vi "Init Power Meter.vi"(8 "error in (no error)":errorcluster, 11 "Application in":refnum<class "Application.lvclass">) -> (0 "error out":errorcluster, 3 "Application out":refnum<class "Application.lvclass">)   [LabVIEW 2018, in "Application.lvlib" / "Application.lvclass"]
uses:
  Application.lvclass
  C:/Program Files/National Instruments/LabVIEW 2018/vi.lib/ActorFramework/Actor/Actor.lvclass
  Application.lvclass/Application.ctl
  User Interface/Splash Screen Messages/Update Status Msg/Update Status Msg.lvclass/Update Status Msg.ctl
  <vilib>/ActorFramework/Message Enqueuer/Message Enqueuer.lvclass/Message Enqueuer.ctl
  <vilib>/ActorFramework/Message Enqueuer/Enqueue.vi
  User Interface/Splash Screen Messages/Update Status Msg/Update Status Msg.lvclass
  C:/Program Files/National Instruments/LabVIEW 2018/vi.lib/ActorFramework/Message/Message.lvclass
  Hardware/Power Meter/Power Meter/Power Meter.lvclass
  <vilib>/ActorFramework/Message Priority Queue/Priority Enqueue.vi
  <vilib>/ActorFramework/Actor/Actor.lvclass
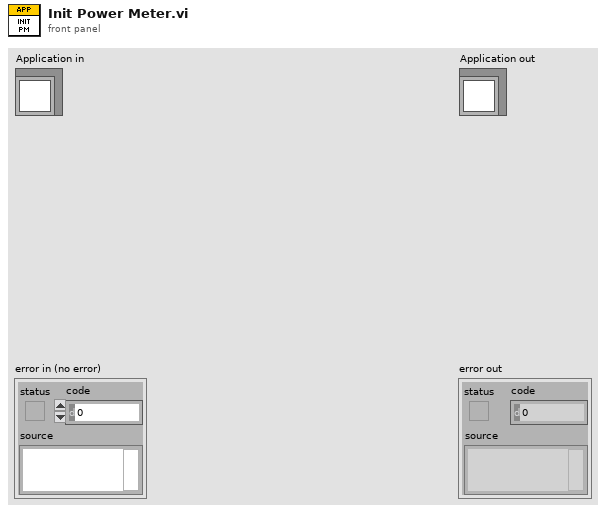
[diagram p1: front panel]
types:
  T1 = enum16{"Disabled", "Thorlabs", "Newport", "Coherent"}
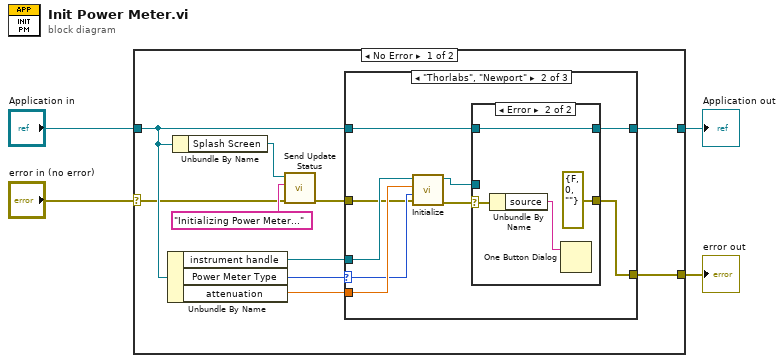
[diagram p0: block diagram]
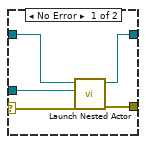
[diagram p3: hidden frame]
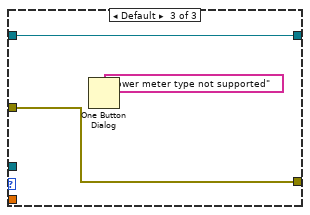
[diagram p4: hidden frame]
diagram:
  n1 = case shown="No Error" "error in (no error)" {
    selector: "error in (no error)" -> [w6 w39]
    tunnel: [w12 w39] -> w3
    tunnel: [w13 w38] -> w1
    tunnel: "Application in" -> [w7 w38]
    frame No Error {
      n2 = Unbundle By Name(w7) -> ("instrument handle"=w10:refnum<visa-resource-name>, "Power Meter Type"=w14:T1, "attenuation"=w11:dbl)
      n3 = Unbundle By Name(w7) -> ("Splash Screen"=w8:refnum<class "Message Enqueuer.lvclass">)
      n4 = call "Send Update Status.vi"("error in (no error)"=w6, "Status Message"="Initializing Power Meter...", "Message Enqueuer"=w8) -> ("error out"=w5:errorcluster)  [unwired: 7 in, 1 out]
      n5 = case shown="\"Thorlabs\", \"Newport\"" w14 {
        selector: w14 -> [_ w19 _]
        tunnel: [w15 w25 w35] -> w12
        tunnel: [w16 w24 w36] -> w13
        tunnel: w7 -> [w16 w18 w36]
        tunnel: w5 -> [w15 w17 w35]
        tunnel: w11 -> [_ w21 _]
        tunnel: w10 -> [_ w20 _]
        frame "Disabled" {
        }
        frame "Thorlabs", "Newport" {
          n6 = call "Initialize.vi"("error in (no error)"=w17, "Power Meter Type"=w19, "attenuation"=w21, "instrument handle"=w20) -> ("error out"=w22:errorcluster, "Power Meter out"=w23:refnum<class "Power Meter.lvclass">)  [unwired: 6 in]
          n7 = case shown="Error" w22 {
            selector: w22 -> [w26 w32]
            tunnel: [w30 errorcluster {"status"=FALSE, "code"=0, "source"=""} ("error out")] -> w25
            tunnel: [w29 w33] -> w24
            tunnel: w18 -> [w28 w33]
            tunnel: w23 -> [w27 _]
            frame No Error {
              n8 = call <vilib>:"Launch Nested Actor.vi"("error in (no error)"=w26, "Nested Actor"=w27, "Caller Actor in"=w28) -> ("error out"=w30:errorcluster, "Caller Actor out"=w29:refnum<class "Application.lvclass">)  [unwired: 6 in, 1 out]
            }
            frame Error {
              n9 = Unbundle By Name(w32) -> ("source"=w31:string)
              n10 = One Button Dialog(message=w31) -> ()  [unwired: 1 in, 1 out]
            }
          }
        }
        frame Default {
          n11 = One Button Dialog(message="Power meter type not supported") -> ()  [unwired: 1 in, 1 out]
        }
      }
    }
    frame Error {
    }
  }
  "error out" <- w3
  "Application out" <- w1
